vi "LSX Set Switch Type.vi"(6 "lAP":i32, 7 "lZP":i32, 8 "error in (no error)":errorcluster, 9 "lYP":i32, 10 "lXP":i32, 11 "lLSID":i32) -> (0 "error out":errorcluster, 3 "function return":i32)   [LabVIEW 2018, in "Tango.lvlib"]
doc: "TANGOAPI int TANGOCALL LSX_SetSwitchType (int lLSID, int lXP, int lYP, int lZP, int lAP);"
uses:
  <userlib>/Tango/Tango.lvlib
  <userlib>/Tango/Tango_DLL.dll
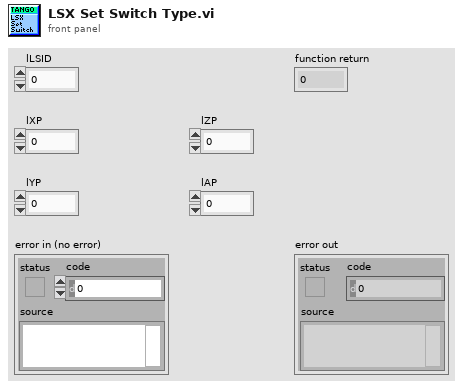
[diagram p1: front panel]
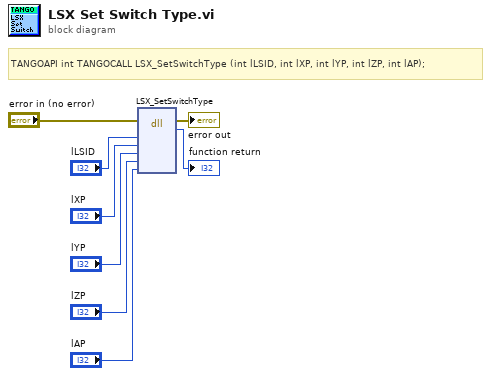
[diagram p0: block diagram]
diagram:
  # "TANGOAPI int TANGOCALL LSX_SetSwitchType (int lLSID, int lXP, int lYP, int lZP, int lAP);"
  n1 = dll-call lib="C:/Program Files (x86)/National Instruments/LabVIEW 2018/user.lib/Tango/Tango_DLL.*" fn="LSX_SetSwitchType"(error in="error in (no error)", "lLSID"="lLSID", "lXP"="lXP", "lYP"="lYP", "lZP"="lZP", "lAP"="lAP") -> (error out=→"error out":errorcluster, →"function return":i32)  [unwired: 7 in, 1 out]
